vi "Append Table.vi"(0 "PDF Report IN":refnum<class "PDF Report Class.lvclass">, 1 "Column Header format":T1={"Cell Type, Alignment and LS"={"Cell Alignment"=5, "Text rotation"=enum."None", "Line spacing"=enum."Select"}, "Font"={"Name"="", "Size"=-1.0, "Color"=0, "Style"={"Bold"=FALSE, "Italic"=FALSE, "Underline"=FALSE, "Strikeout"=FALSE}, "Type"={"Type&direction"=enum."Select", "Embedded"=FALSE, "Encoding"=""}}}, 2 "Predefined Borders":T18={"Borders"=1, "Header"={"Thickness"=1.0, "Line"=0, "Background "=16777215}, "Data"={"Thickness"=0.5, "Line"=0, "Background "=16777215}}, 3 "Row background color":T20={"color"=16777225, "at each"=0}, 5 "Table properties":T11={"Table position"=1, "SpacingBefore (points)"=0.0, "SpacingAfter (points)"=0.0} {"Table position" items=["LEFT", "CENTER", "RIGHT"]}, 7 "PDF Table":refnum<class "Pdfp Table Class.lvclass">, 9 "Caption":string, 11 "error in (no error)":errorcluster, 12 "Row Header format":T1={"Cell Type, Alignment and LS"={"Cell Alignment"=5, "Text rotation"=enum."None", "Line spacing"=enum."Select"}, "Font"={"Name"="", "Size"=-1.0, "Color"=0, "Style"={"Bold"=FALSE, "Italic"=FALSE, "Underline"=FALSE, "Strikeout"=FALSE}, "Type"={"Type&direction"=enum."Select", "Embedded"=FALSE, "Encoding"=""}}}, 13 "Datas format":T1={"Cell Type, Alignment and LS"={"Cell Alignment"=5, "Text rotation"=enum."None", "Line spacing"=enum."Select"}, "Font"={"Name"="", "Size"=-1.0, "Color"=0, "Style"={"Bold"=FALSE, "Italic"=FALSE, "Underline"=FALSE, "Strikeout"=FALSE}, "Type"={"Type&direction"=enum."Select", "Embedded"=FALSE, "Encoding"=""}}}, 14 "Custom Table Borders":T13) -> (4 "PDF Report OUT":refnum<class "PDF Report Class.lvclass">, 15 "error out":errorcluster)   [LabVIEW 2020, in "Exaprom PDF.lvlib"]
doc: "<B>ENGLISH</B>\nAppends a table to the PDF document.\n\n<B>FRANÇAIS</B>\nAjoute un tableau au document PDF.\n\nDeveloped by Jean-Marc Simard\nCopyright © 2011, Exaprom Inc.\nAll rights reserved.\nLicense: BSD\n\nWith iTextSharp 4.1.6 (http://itextsharp.sourceforge.net)\nunder Mozilla Public License Version 1.1\n(http://www.mozilla.org/MPL/MPL-1.1.html)"
uses:
  <userlib>/labview-PDF-writer-master/Exaprom PDF.lvlib
  <userlib>/labview-PDF-writer-master/LV Class/PDF Report Class/PDF Report Class.lvclass
  <userlib>/labview-PDF-writer-master/Controls/Table Controls/Row Back Ground color Datas.ctl
  <userlib>/labview-PDF-writer-master/LV Class/Pdfp Table Class/Pdfp Table Class.lvclass
  <userlib>/labview-PDF-writer-master/Controls/Table Controls/Row Predefined borders cluster.ctl
  <userlib>/labview-PDF-writer-master/Controls/Table Controls/Row Predefined borders.ctl
  <userlib>/labview-PDF-writer-master/Controls/Table Controls/Simplified Table Row Borders [ ].ctl
  <userlib>/labview-PDF-writer-master/Controls/Table Controls/Simplified Table Row Borders.ctl
  <userlib>/labview-PDF-writer-master/Controls/Table Controls/Border and BG Color [ ].ctl
  <userlib>/labview-PDF-writer-master/Controls/Table Controls/Border and BG Color.ctl
  <userlib>/labview-PDF-writer-master/Controls/Table Controls/Cell Border 20 px.ctl
  <userlib>/labview-PDF-writer-master/Controls/Table Controls/Cell Font, type, Alignment and LS V2.ctl
  <userlib>/labview-PDF-writer-master/Controls/Table Controls/Cell Type, Alignment and LS.ctl
  <userlib>/labview-PDF-writer-master/Controls/Table Controls/Cell Alignment 20px.ctl
  <userlib>/labview-PDF-writer-master/Controls/Table Controls/Text vertical arrangement.ctl
  <userlib>/labview-PDF-writer-master/Controls/Text Controls/Line spacing.ctl
  <userlib>/labview-PDF-writer-master/Controls/Font Controls/Font complete cluster.ctl
  <userlib>/labview-PDF-writer-master/Controls/Font Controls/Font size.ctl
  <userlib>/labview-PDF-writer-master/Controls/Font Controls/Font color.ctl
  <userlib>/labview-PDF-writer-master/Controls/Font Controls/Type and encoding.ctl
  <userlib>/labview-PDF-writer-master/Controls/Text Controls/Unicode/Type and run direction.ctl
  <userlib>/labview-PDF-writer-master/Controls/Table Controls/Table properties.ctl
  <userlib>/labview-PDF-writer-master/Controls/Table Controls/Table position.ctl
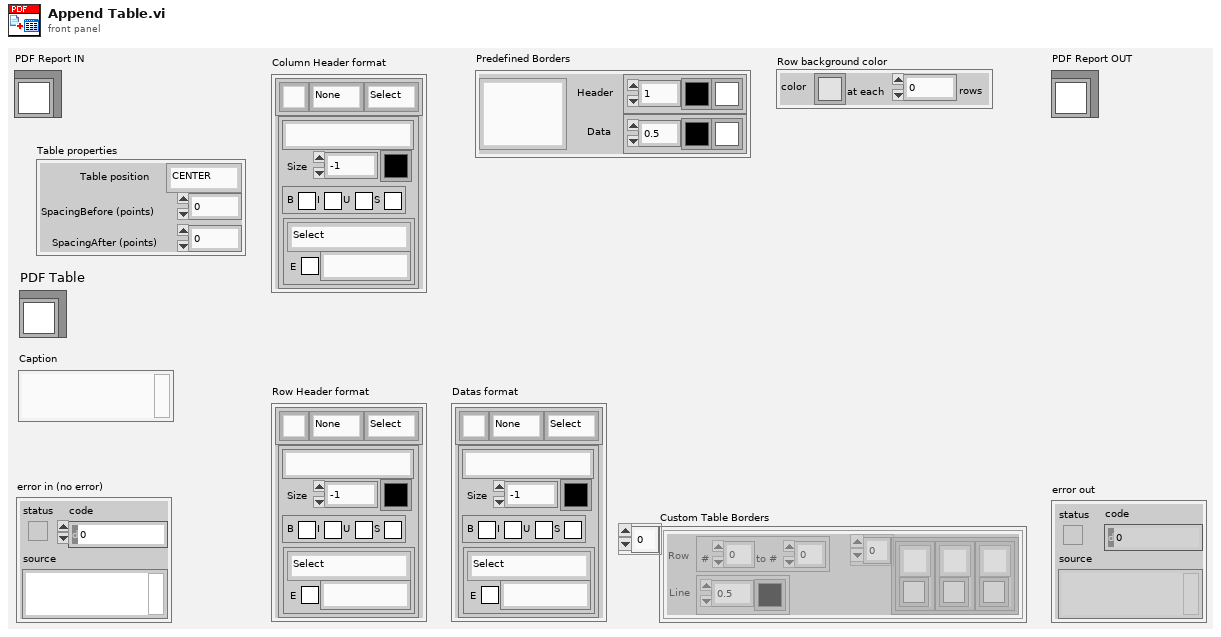
[diagram p1: front panel]
types:
  T1 = typedef "Exaprom PDF.lvlib/Cell Font, type, Alignment and LS V2.ctl" = cluster{"Cell Type, Alignment and LS":T2, "Font":T6}
  T2 = typedef "Exaprom PDF.lvlib/Cell Type, Alignment and LS.ctl" = cluster{"Cell Alignment":T3, "Text rotation":T4, "Line spacing":T5}
  T3 = typedef "Exaprom PDF.lvlib/Cell Alignment 20px.ctl" = u16
  T4 = typedef "Exaprom PDF.lvlib/Text vertical arrangement.ctl" = enum16{"None", "Clockwise", "Counterclockwise"}
  T5 = typedef "Exaprom PDF.lvlib/Line spacing.ctl" = enum16{"Select", "1.0", "1.5", "2.0"}
  T6 = typedef "Exaprom PDF.lvlib/Font complete cluster.ctl" = cluster{"Name":string, "Size":T7, "Color":T8, "Style":cluster{"Bold":bool, "Italic":bool, "Underline":bool, "Strikeout":bool}, "Type":T9}
  T7 = typedef "Exaprom PDF.lvlib/Font size.ctl" = sgl
  T8 = typedef "Exaprom PDF.lvlib/Font color.ctl" = u32
  T9 = typedef "Exaprom PDF.lvlib/Type and encoding.ctl" = cluster{"Type&direction":T10, "Embedded":bool, "Encoding":string}
  T10 = typedef "Exaprom PDF.lvlib/Type and run direction.ctl" = enum16{"Select", "ASCII", "UTF-16", "UTF-16 (default)", "UTF-16 (LTR)", "UTF-16 (RTL)"}
  T11 = typedef "Exaprom PDF.lvlib/Table properties.ctl" = cluster{"Table position":T12, "SpacingBefore (points)":sgl, "SpacingAfter (points)":sgl}
  T12 = typedef "Exaprom PDF.lvlib/Table position.ctl" = i32
  T13 = typedef "Exaprom PDF.lvlib/Simplified Table Row Borders [ ].ctl" = T14[]
  T14 = typedef "Exaprom PDF.lvlib/Simplified Table Row Borders.ctl" = cluster{"Row":cluster{"#":i16, "to #":i16}, "Line":cluster{"Thickness":sgl, "Color":u32}, "Column Borders [ ]":T15}
  T15 = typedef "Exaprom PDF.lvlib/Border and BG Color [ ].ctl" = T16[]
  T16 = typedef "Exaprom PDF.lvlib/Border and BG Color.ctl" = cluster{"Cell Border":T17, "BG":u32}
  T17 = typedef "Exaprom PDF.lvlib/Cell Border 20 px.ctl" = u16
  T18 = typedef "Exaprom PDF.lvlib/Row Predefined borders cluster.ctl" = cluster{"Borders":T19, "Header":cluster{"Thickness":sgl, "Line":u32, "Background ":u32}, "Data":cluster{"Thickness":sgl, "Line":u32, "Background ":u32}}
  T19 = typedef "Exaprom PDF.lvlib/Row Predefined borders.ctl" = u16
  T20 = typedef "Exaprom PDF.lvlib/Row Back Ground color Datas.ctl" = cluster{"color":u32, "at each":i16}
  T21 = typedef "Exaprom PDF.lvlib/Table Appearance and Font Row [ ].ctl" = T22[]
  T22 = typedef "Exaprom PDF.lvlib/One Row Appearance.ctl" = cluster{"Row":T23, "Cell [ ]":T24[]}
  T23 = typedef "Exaprom PDF.lvlib/Row from to.ctl" = cluster{"From #":i16, "to #":i16}
  T24 = typedef "Exaprom PDF.lvlib/Cell, Alignment, LS and Font - hide Vmerge.ctl" = cluster{"Text":T2, "Cell Appearance":T25, "HMerge":T26, "VMerge":T27, "Font":T6}
  T25 = typedef "Exaprom PDF.lvlib/Cell Appearance.ctl" = cluster{"Border":T17, "Thickness":sgl, "Color":u32, "BG":u32}
  T26 = typedef "Exaprom PDF.lvlib/Merge Horizontal.ctl" = cluster{"From":i8, "to":i8}
  T27 = typedef "Exaprom PDF.lvlib/Merge Vertical.ctl" = cluster{"From":i8, "to":i8}
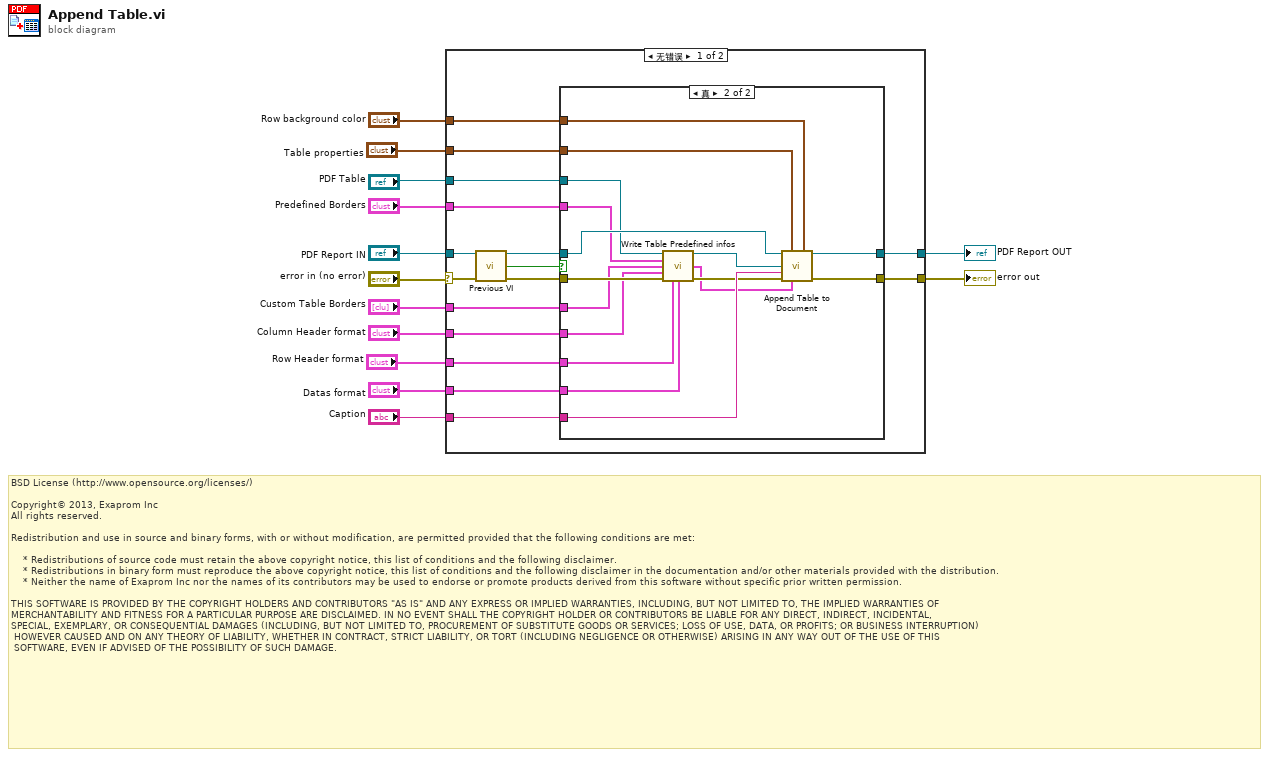
[diagram p0: block diagram]
diagram:
  # "BSD License (http://www.opensource.org/licenses/)\n\nCopyright© 2013, Exaprom Inc\nAll rights reserved.\n\nRedistribution and use in source and binary forms, with or without modification, are permitted provided that the following conditions are met:\n\n    * Redistributions of source code must retain the above copyright notice, this list of conditions and the following disclaimer.\n    * Redistributions in binary form must reproduce the above copyright notice, this list of conditions and the following disclaimer in the documentation and/or other materials provided with the distribution.\n    * Neither the name of Exaprom Inc nor the names of its contributors may be used to endorse or promote products derived from this software without specific prior written permission.\n\nTHIS SOFTWARE IS PROVIDED BY THE COPYRIGHT HOLDERS AND CONTRIBUTORS \"AS IS\" AND ANY EXPRESS OR IMPLIED WARRANTIES, INCLUDING, BUT NOT LIMITED TO, THE IMPLIED WARRANTIES OF \nMERCHANTABILITY AND FITNESS FOR A PARTICULAR PURPOSE ARE DISCLAIMED. IN NO EVENT SHALL THE COPYRIGHT HOLDER OR CONTRIBUTORS BE LIABLE FOR ANY DIRECT, INDIRECT, INCIDENTAL,\nSPECIAL, EXEMPLARY, OR CONSEQUENTIAL DAMAGES (INCLUDING, BUT NOT LIMITED TO, PROCUREMENT OF SUBSTITUTE GOODS OR SERVICES; LOSS OF USE, DATA, OR PROFITS; OR BUSINESS INTERRUPTION)\n HOWEVER CAUSED AND ON ANY THEORY OF LIABILITY, WHETHER IN CONTRACT, STRICT LIABILITY, OR TORT (INCLUDING NEGLIGENCE OR OTHERWISE) ARISING IN ANY WAY OUT OF THE USE OF THIS\n SOFTWARE, EVEN IF ADVISED OF THE POSSIBILITY OF SUCH DAMAGE."
  n1 = case shown="无错误" "error in (no error)" {
    selector: "error in (no error)" -> [w25 w48]
    tunnel: "PDF Report IN" -> [w23 w49]
    tunnel: "Caption" -> [w29 _]
    tunnel: "Row background color" -> [w28 _]
    tunnel: [w27 w49] -> w9
    tunnel: [w26 w48] -> w8
    tunnel: "PDF Table" -> [w21 _]
    tunnel: "Predefined Borders" -> [w20 _]
    tunnel: "Custom Table Borders" -> [w19 _]
    tunnel: "Column Header format" -> [w18 _]
    tunnel: "Datas format" -> [w17 _]
    tunnel: "Table properties" -> [w16 _]
    tunnel: "Row Header format" -> [w15 _]
    frame No Error {
      n2 = call <userlib>:"Previous VI.vi"("PDF Report IN"=w23, "error in (no error)"=w25) -> ("PDF Report OUT"=w22:refnum<class "PDF Report Class.lvclass">, "Execute Actual VI"=w14:bool, "error out"=w24:errorcluster)  [unwired: 11 out]
      n3 = case shown="真" w14 {
        tunnel: w29 -> [_ w44]
        tunnel: w28 -> [_ w45]
        tunnel: [w31 w46] -> w27
        tunnel: [w30 w47] -> w26
        tunnel: w24 -> [w30 w41]
        tunnel: w22 -> [w31 w43]
        tunnel: w21 -> [_ w38]
        tunnel: w20 -> [_ w40]
        tunnel: w19 -> [_ w39]
        tunnel: w18 -> [_ w35]
        tunnel: w17 -> [_ w33]
        tunnel: w16 -> [_ w36]
        tunnel: w15 -> [_ w34]
        frame False {
        }
        frame True {
          n4 = call <userlib>:"Write Table Predefined infos.vi"("PDF Table Class.lvclass in"=w38, "Predefined Borders"=w40, "Borders IN"=w39, "Column Header format"=w35, "error in (no error)"=w41, "Row Header format"=w34, "Datas format"=w33) -> ("PDF Table Class.lvclass out"=w37:refnum<class "Pdfp Table Class.lvclass">, "Row  [ ] OUT"=w32:T21, "error out"=w42:errorcluster)  [unwired: 6 in]
          n5 = call <userlib>:"Append Table to Document.vi"("PDF Report IN"=w43, "Table properties"=w36, "Row background color"=w45, "PDF Table"=w37, "Caption"=w44, "error in (no error)"=w42, "Row  [ ]"=w32) -> ("PDF Report OUT"=w46:refnum<class "PDF Report Class.lvclass">, "error out"=w47:errorcluster)  [unwired: 7 out]
        }
      }
    }
    frame Error {
    }
  }
  "error out" <- w8
  "PDF Report OUT" <- w9
